vi "sub_receive_parsing.vi"(8 "error in":errorcluster caption="err-in", 11 "data_out 입력":string) -> (0 "error out":errorcluster caption="err-out")   [LabVIEW 2017]
panel:
  out "str_steer":string
  out "st":i16
  out "sp":i16
  out "str_speed":string
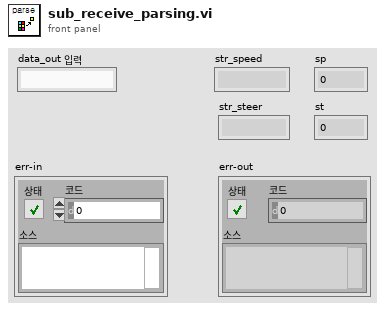
[diagram p1: front panel]
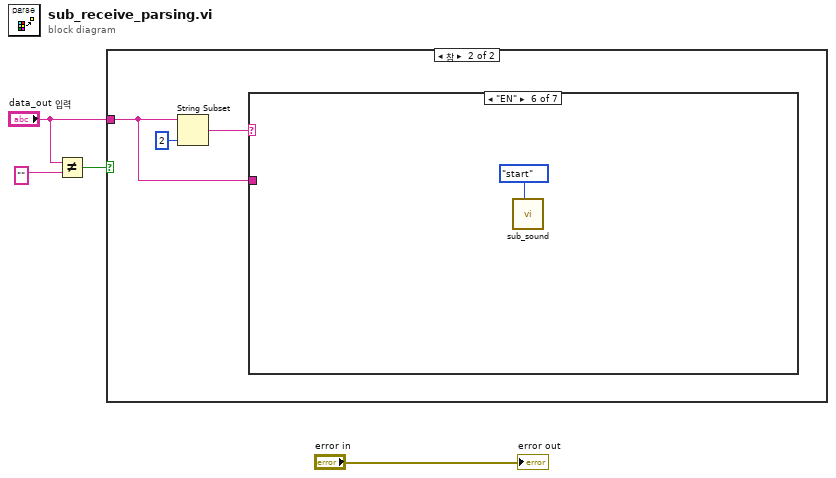
[diagram p0: block diagram]
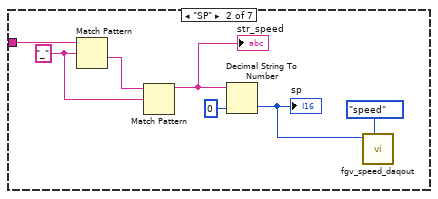
[diagram p4: hidden frame]
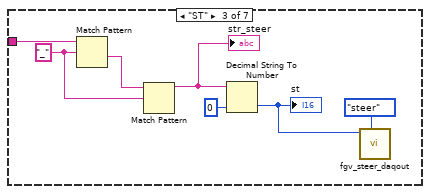
[diagram p5: hidden frame]
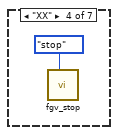
[diagram p6: hidden frame]
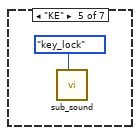
[diagram p7: hidden frame]
diagram:
  n1 = Not Equal?(x="data_out 입력", y="" ("data_out 2")) -> (x != y?=w3:bool)
  n2 = case shown="참" w3 {
    tunnel: "data_out 입력" -> [_ w5]
    frame False {
    }
    frame True {
      n3 = String Subset(string=w5, length (rest)=2 ("길이(나머지)")) -> (substring=w6:string)  [unwired: 1 in]
      n4 = case shown="\"EN\"" w6 {
        tunnel: w5 -> [_ w14 w21 _ _ _ _]
        frame "거짓", Default {
        }
        frame "SP" {
          w12 = "_" ("정규식")
          n5 = Match Pattern(string=w14, regular expression=w12) -> (after substring=w13:string)  [unwired: 1 in, 3 out]
          n6 = Match Pattern(string=w13, regular expression=w12) -> (before substring=w11:string)  [unwired: 1 in, 3 out]
          "str_speed" <- w11
          n7 = Decimal String To Number(string=w11, default (0L)=i16 0 ("기본(0 I32)")) -> (number=w9:i16)  [unwired: 1 in, 1 out]
          "sp" <- w9
          n8 = call "fgv_speed_daqout.vi"("cmd"=enum16{"speed", "close", "ini"}."speed", "speed"=w9) -> ()  [unwired: 9 in, 1 out]
        }
        frame "ST" {
          w19 = "_" ("정규식")
          n9 = Match Pattern(string=w21, regular expression=w19) -> (after substring=w20:string)  [unwired: 1 in, 3 out]
          n10 = Match Pattern(string=w20, regular expression=w19) -> (before substring=w18:string)  [unwired: 1 in, 3 out]
          "str_steer" <- w18
          n11 = Decimal String To Number(string=w18, default (0L)=i16 0 ("기본(0 I32)")) -> (number=w16:i16)  [unwired: 1 in, 1 out]
          "st" <- w16
          n12 = call "fgv_steer_daqout.vi"("cmd"=enum16{"steer", "close", "ini"}."steer", "steer"=w16) -> ()  [unwired: 9 in, 1 out]
        }
        frame "XX" {
          n13 = call "fgv_stop.vi"("cmd"=enum16{"default", "ini", "stop"}."stop") -> ()  [unwired: 9 in, 2 out]
        }
        frame "KE" {
          n14 = call "sub_sound.vi"("cmd"=enum16{"start", "key_lock"}."key_lock") -> ()  [unwired: 10 in, 1 out]
        }
        frame "EN" {
          n15 = call "sub_sound.vi"("cmd"=enum16{"start", "key_lock"}."start") -> ()  [unwired: 10 in, 1 out]
        }
        frame "-" {
        }
      }
    }
  }
  "error out" <- "error in"
